vi "ParseRenameInfo.vi"(8 "error in (no error)":errorcluster) -> (0 "error out":errorcluster, 3 "Rename Info":T1)   [LabVIEW 2024]
uses:
  RenameInfo.ctl
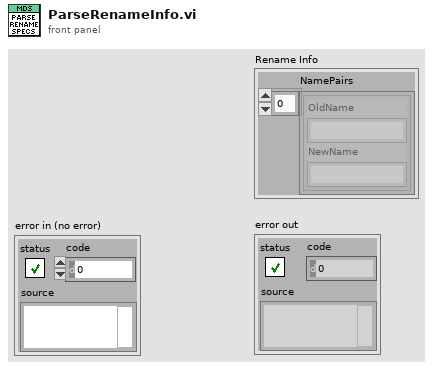
[diagram p1: front panel]
types:
  T1 = typedef "RenameInfo.ctl" = cluster{"NamePairs":cluster{"OldName":string, "NewName":string}[]}
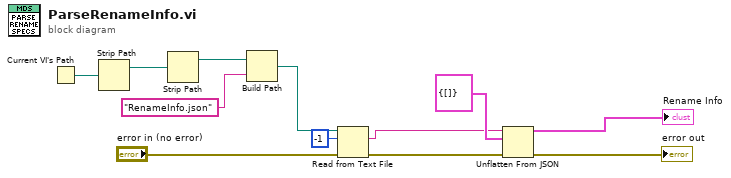
[diagram p0: block diagram]
diagram:
  n1 = Current VI's Path() -> (path=w12:path)
  n2 = Strip Path(path=w12) -> (stripped path=w2:path)  [unwired: 1 out]
  n3 = Strip Path(path=w2) -> (stripped path=w1:path)  [unwired: 1 out]
  n4 = Build Path(base path=w1, name or relative path="RenameInfo.json" ("pattern")) -> (appended path=w5:path)
  n5 = Read from Text File(file (use dialog)=w5, count=-1, error in="error in (no error)") -> (text=w7:string, error out=w8:errorcluster)  [unwired: 1 in, 2 out]
  n6 = Unflatten From JSON(JSON string=w7, type and defaults=T1 {"NamePairs"=[]} ("Rename Spec"), error in (no error)=w8) -> (value=→"Rename Info":T1, error out=→"error out":errorcluster)  [unwired: 4 in]
